vi "Autonomous_Thread.vi"() -> ()   [LabVIEW 2014]
doc: "This VI is called when autonomous begins, and will automatically be terminated when autonomous ends. You can carry out timed or sensor driven robot movement independently without needing to return to the caller."
uses:
  <vilib>/Rock Robotics/Network Tables/SD Write String.vi
  Auto_Conf.vi
panel:
  in  "Automodes":string[](array[string])=["auto_0.bee", "auto_1.bee", "auto_2.bee", "auto_3.bee", "auto_4.bee", "auto_5.bee", "auto_6.bee", "auto_7.bee"]
  # "Each item in this array is an autonomous script file.\nThis array is indexed by the autoMode variable in Robot Global Data."
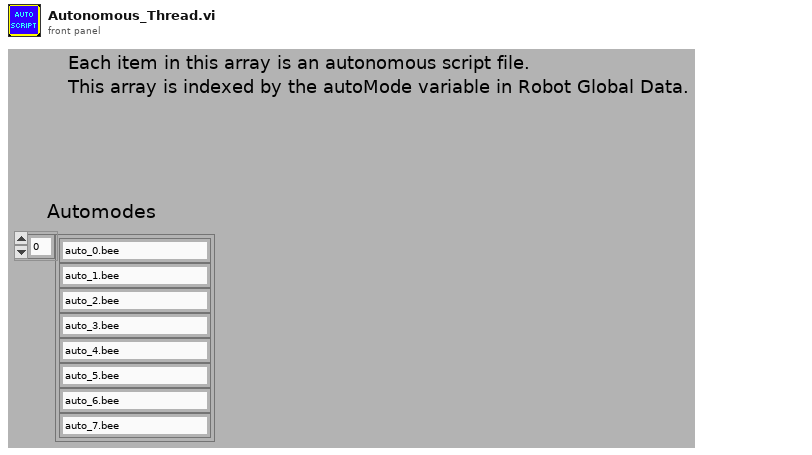
[diagram p1: front panel]
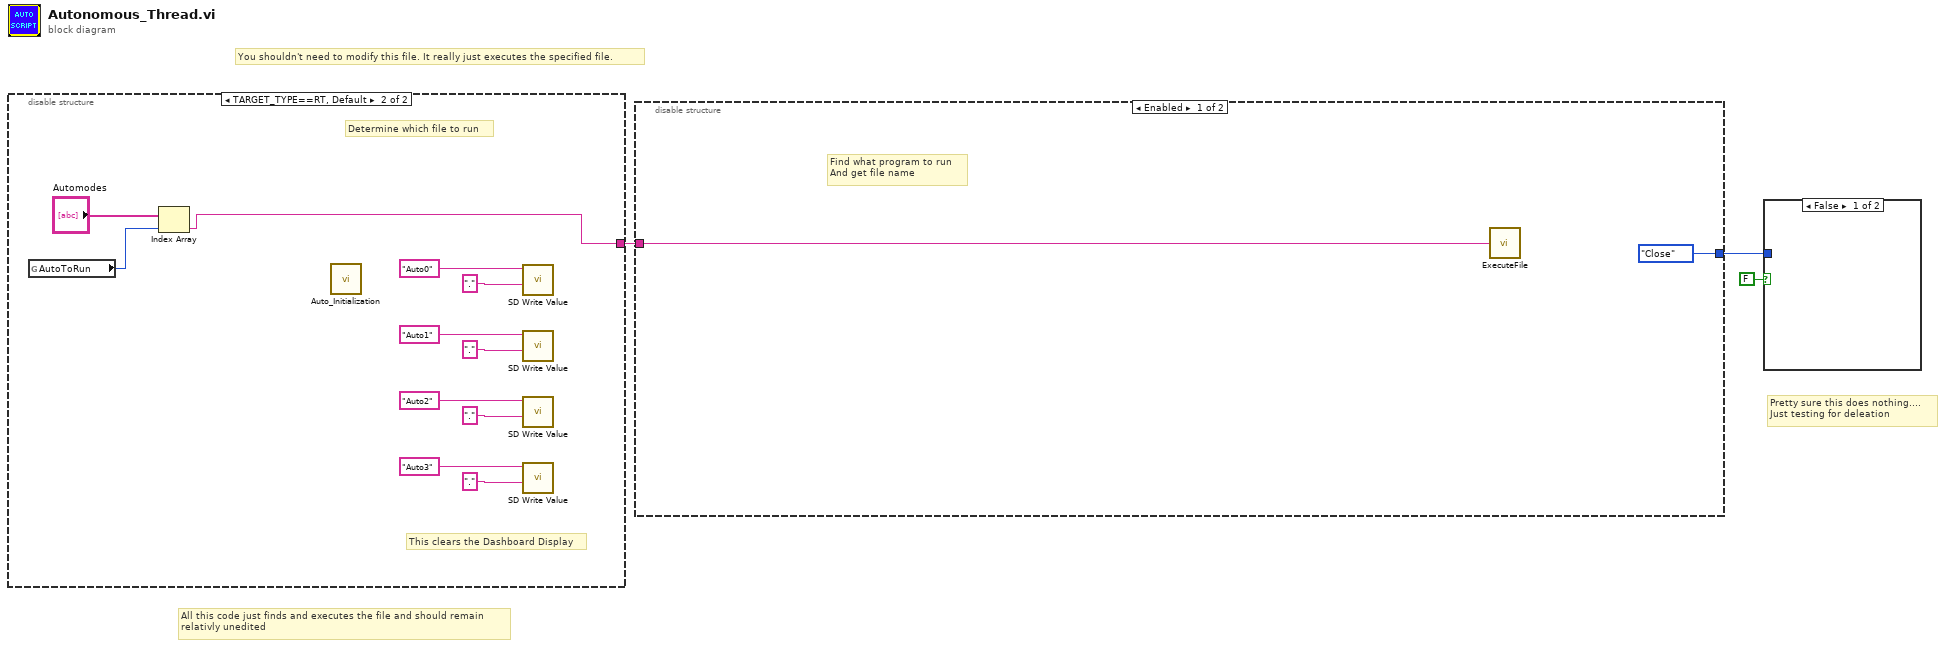
[diagram p0: block diagram]
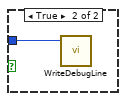
[diagram p2: hidden frame]
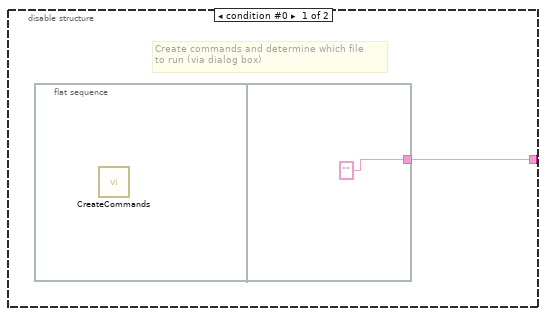
[diagram p3: hidden frame]
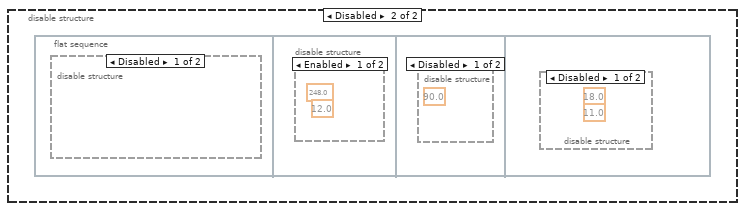
[diagram p4: hidden frame]
diagram:
  # "Pretty sure this does nothing.... \nJust testing for deleation"
  # "All this code just finds and executes the file and should remain\nrelativly unedited"
  # "You shouldn't need to modify this file. It really just executes the specified file."
  n1 = disable-structure shown="TARGET_TYPE==RT, Default" {
    disable-tunnel: [w4 w15] -> w3
    frame condition #0 {
      # "Create commands and determine which file\nto run (via dialog box)"
      n2 = flat-sequence {
        tunnel: ["" ("File Name With Extension")] -> w4
        frame #0 {
          n3 = call "CreateCommands.vi"() -> ()  [unwired: 1 out]
        }
        frame #1 {
        }
      }
    }
    frame condition #1 (active) {
      # "This clears the Dashboard Display"
      # "Determine which file to run"
      n4 = global read "Auto_Conf.vi" "AutoToRun"() -> (w14:u8)
      n5 = Index Array(array="Automodes", index=w14) -> (element=w15:string)
      n6 = call "Auto_Initialization.vi"() -> ()  [unwired: 1 in]
      n7 = call-poly <vilib>:"SD Write Value.vi"("String"=".", "Name"="Auto0") -> ()  [unwired: 8 in, 2 out]
      n8 = call-poly <vilib>:"SD Write Value.vi"("String"=".", "Name"="Auto1") -> ()  [unwired: 8 in, 2 out]
      n9 = call-poly <vilib>:"SD Write Value.vi"("String"=".", "Name"="Auto2") -> ()  [unwired: 8 in, 2 out]
      n10 = call-poly <vilib>:"SD Write Value.vi"("String"=".", "Name"="Auto3") -> ()  [unwired: 8 in, 2 out]
    }
  }
  n11 = disable-structure shown="Enabled" {
    disable-tunnel: w3 -> [w18 _]
    disable-tunnel: [enum16{"Open", "Write Line", "Close"}."Close" ("Mode") _] -> w2
    frame Enabled {
      # "Find what program to run\nAnd get file name"
      n12 = call "ExecuteFile.vi"("File Name With Extension"=w18) -> ()
    }
    frame Disabled {
      n13 = flat-sequence {
        frame #0 {
          n14 = disable-structure shown="Disabled" {
            frame Disabled {
            }
            frame Enabled {
            }
          }
        }
        frame #1 {
          n15 = disable-structure shown="Enabled" {
            frame Enabled {
              (unwired) 248.0 ("Distance")
              (unwired) 12.0 ("Speed (ft/sec)")
            }
            frame Disabled {
            }
          }
        }
        frame #2 {
          n16 = disable-structure shown="Disabled" {
            frame Disabled {
              (unwired) 90.0 ("Angle")
            }
            frame Enabled {
            }
          }
        }
        frame #3 {
          n17 = disable-structure shown="Disabled" {
            frame Disabled {
              (unwired) 18.0 ("Distance")
              (unwired) 11.0 ("Speed (ft/sec)")
            }
            frame Enabled {
            }
          }
        }
      }
    }
  }
  n18 = case shown="False" FALSE {
    tunnel: w2 -> [_ w19]
    frame False {
    }
    frame True {
      n19 = call "WriteDebugLine.vi"("Mode"=w19) -> ()  [unwired: 1 in, 10 out]
    }
  }
